vi "AudioStreamer.Validate Configuration.vi"(0 "config":T1) -> (4 "config thru":T1, 15 "error out":errorcluster)   [LabVIEW 2020]
uses:
  Typedefs/AudioStreamer.Config.ctl
  Typedefs/AudioStreamer.Signal Specification.ctl
  <vilib>/Dataflow_G/G-Audio/Controls/Audio Device Format.ctl
  <vilib>/Utility/error.llb/Error Cluster From Error Code.vi
  <vilib>/ErrorRing/Error Ring.xnode
  <vilib>/Dataflow_G/G-Audio/G-Audio.lvlib
panel:
  in  "Format":T3=enum."SGL"
  in  "Channels":u32=8
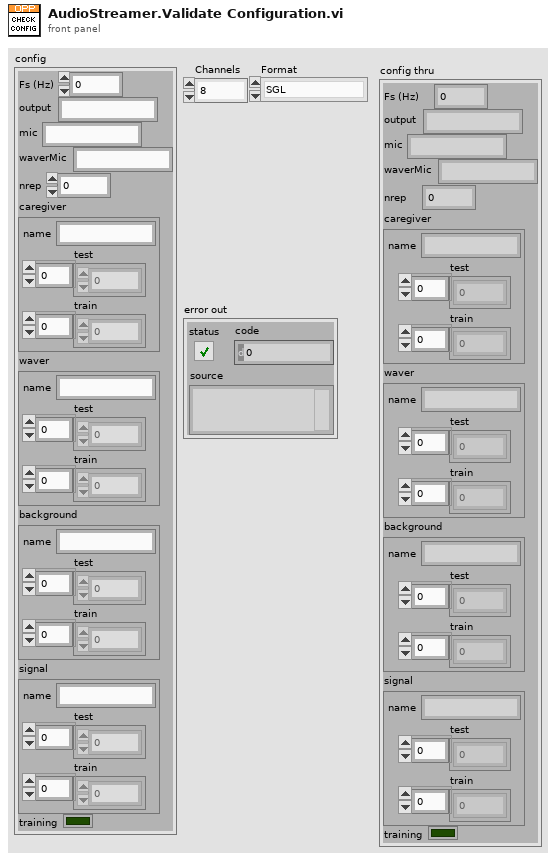
[diagram p1: front panel]
types:
  T1 = typedef "AudioStreamer.Config.ctl" = cluster{"Fs (Hz)":dbl, "output":string, "mic":string, "waverMic":string, "nrep":i32, "caregiver":T2, "waver":T2, "background":T2, "signal":T2, "training":bool}
  T2 = typedef "AudioStreamer.Signal Specification.ctl" = cluster{"name":string, "test":sgl[], "train":sgl[]}
  T3 = typedef "G-Audio.lvlib/Audio Device Format.ctl" = enum16{"Native", "U8", "I16", "I32", "SGL"}
  T4 = typedef "G-Audio.lvlib/Audio Device Info.ctl" = cluster{"Name":string, "ID":u8[], "Device Type":T5, "Default":bool, "Native Data Formats":T6[]}
  T5 = typedef "G-Audio.lvlib/Audio Device Type.ctl" = enum16{"(None)", "Playback", "Capture", "Duplex", "Loopback"}
  T6 = typedef "G-Audio.lvlib/Audio Device Native Data Format.ctl" = cluster{"Format":T3, "Channels":u32, "Sample Rate (Hz)":u32, "Exclusive Mode":bool}
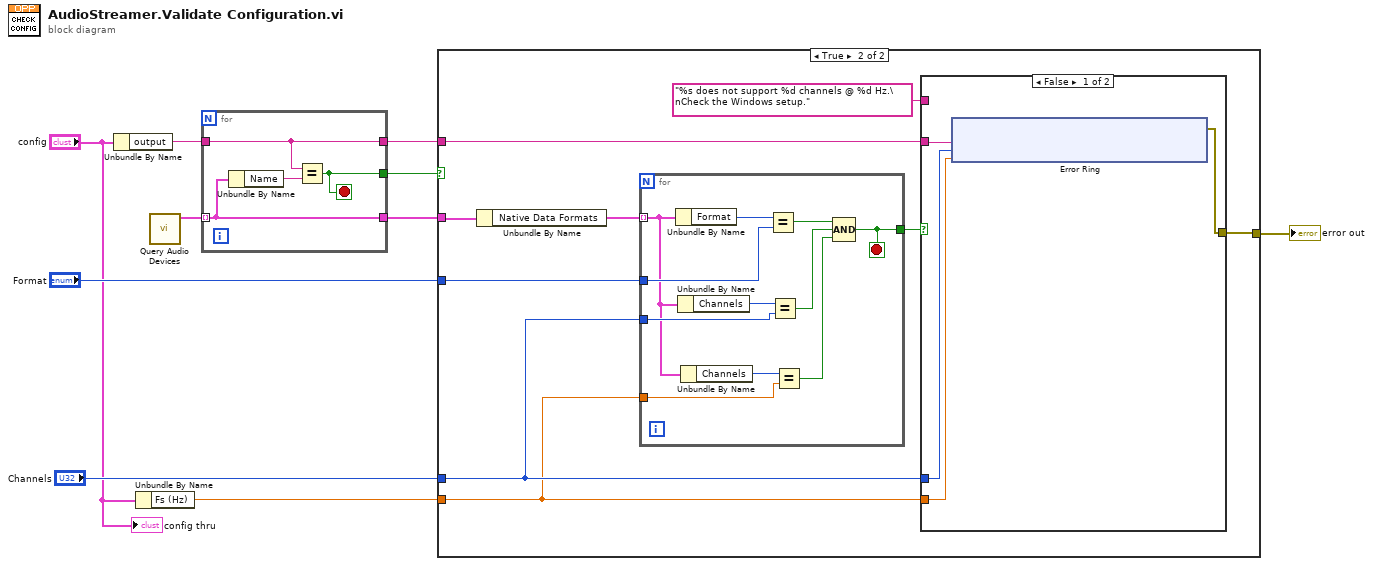
[diagram p0: block diagram]
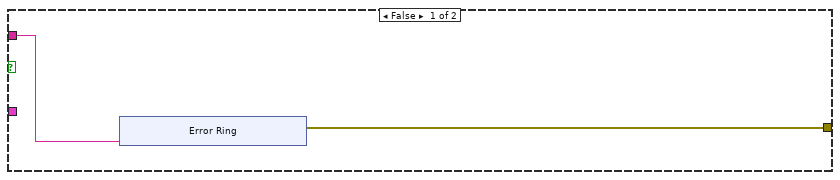
[diagram p2: hidden frame]
diagram:
  n1 = Unbundle By Name("config") -> ("output"=w10:string)
  n2 = Unbundle By Name("config") -> ("Fs (Hz)"=w2:dbl)
  n3 = call <vilib>:"Query Audio Devices.vi"() -> ("Playback Devices"=w9:T4[])  [unwired: 7 in, 4 out]
  n4 = for {
    tunnel: w10 -> [w14]
    tunnel: [w14] -> w6
    tunnel: w9 -> [w12] mode=indexing
    tunnel: [w12] -> w7
    tunnel: [w11] -> w8
    stop <- w11 stop-if-true
    n5 = Unbundle By Name(w12) -> ("Name"=w13:string)
    n6 = Equal?(x=w14, y=w13) -> (x = y?=w11:bool)
  }
  n7 = case shown="True" w8 {
    tunnel: [w15 w24] -> w1
    tunnel: w6 -> [w16 w28]
    tunnel: w7 -> [_ w32]
    tunnel: "Format" -> [_ w30]
    tunnel: "Channels" -> [_ w26]
    tunnel: w2 -> [_ w25]
    frame False {
      n8 = xnode "Error Ring"("parameter 0"=w16) -> ("error out"=w15:errorcluster)
    }
    frame True {
      n9 = Unbundle By Name(w32) -> ("Native Data Formats"=w31:T6[])
      n10 = for {
        tunnel: w31 -> [w52] mode=indexing
        tunnel: w30 -> [w55]
        tunnel: w26 -> [w53]
        tunnel: w25 -> [w51]
        tunnel: [w46] -> w29
        stop <- w46 stop-if-true
        n11 = Unbundle By Name(w52) -> ("Format"=w56:T3)
        n12 = Unbundle By Name(w52) -> ("Channels"=w54:u32)
        n13 = Unbundle By Name(w52) -> ("Channels"=w50:u32)
        n14 = Equal?(x=w56, y=w55) -> (x = y?=w49:bool)
        n15 = Equal?(x=w54, y=w53) -> (x = y?=w48:bool)
        n16 = Equal?(x=w50, y=w51) -> (x = y?=w47:bool)
        n17 = Compound Arithmetic op=AND(w49, w48, w47) -> (w46:bool)
      }
      n18 = case shown="False" w29 {
        tunnel: w28 -> [w36 _]
        tunnel: "%s does not support %d channels @ %d Hz.\nCheck the Windows setup." ("format string") -> [_ _]
        tunnel: w26 -> [w35 _]
        tunnel: w25 -> [w34 _]
        tunnel: [w33 _] -> w24
        frame False {
          n19 = xnode "Error Ring"("parameter 0"=w36, "parameter 1"=w35, "parameter 2"=w34) -> ("error out"=w33:errorcluster)
        }
        frame True {
        }
      }
    }
  }
  "error out" <- w1
  "config thru" <- "config"
